vi "rotateArray.vi"(6 "Rotate":i32, 8 "Array in":u16[](array[numeric]) format="%016b") -> (3 "Array out":u16[](array[numeric]) format="%016b")   [LabVIEW 2013]
doc: "Rotates elements in array"
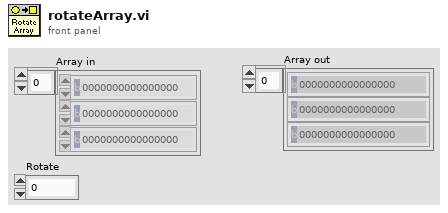
[diagram p1: front panel]
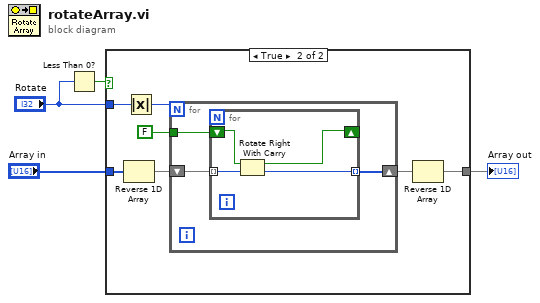
[diagram p0: block diagram]
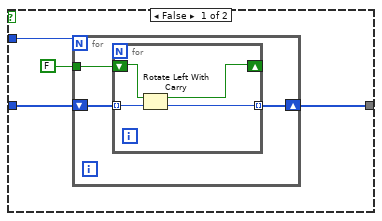
[diagram p2: hidden frame]
diagram:
  n1 = Less Than 0?(x="Rotate") -> (x < 0?=w1:bool)
  n2 = case shown="True" w1 {
    tunnel: "Array in" -> [w7 w21]
    tunnel: [w6 w17] -> w3
    tunnel: "Rotate" -> [w5 w20]
    frame False {
      n3 = for {
        N: w5 -> [_]
        shift-right: [w10] -> w6
        shift-left: w7 -> [w11]
        tunnel: FALSE ("msb carry out") -> [w9]
        n4 = for {
          shift-right: [w12] -> _
          shift-left: w9 -> [w13]
          tunnel: w11 -> [w15] mode=indexing
          tunnel: [w14] -> w10 mode=indexing
          n5 = Rotate Left With Carry(2:w15, 3:w13) -> (0:w14:u16, 1:w12:bool)
        }
      }
    }
    frame True {
      n6 = Reverse 1D Array(array=w21) -> (reversed array=w19:u16[])
      n7 = Absolute Value(x=w20) -> (abs(x)=w16:i32)
      n8 = for {
        N: w16 -> [_]
        shift-right: [w24] -> w18
        shift-left: w19 -> [w25]
        tunnel: FALSE ("msb carry out") -> [w23]
        n9 = for {
          shift-right: [w26] -> _
          shift-left: w23 -> [w27]
          tunnel: w25 -> [w29] mode=indexing
          tunnel: [w28] -> w24 mode=indexing
          n10 = Rotate Right With Carry(2:w29, 3:w27) -> (0:w28:u16, 1:w26:bool)
        }
      }
      n11 = Reverse 1D Array(array=w18) -> (reversed array=w17:u16[])
    }
  }
  "Array out" <- w3
